vi "Waveform Analysis (Polling).vi"() -> ()   [LabVIEW 2012]
uses:
  <vilib>/Analysis/2dsp.llb/Real FFT.vi
  <vilib>/Analysis/NI_AALPro.lvlib
panel:
  out "频谱":dbl[](graph)
  out "最小值":dbl
  out "最大值":dbl
  out "时间序列":dbl[](graph)
  in  "获取最大值与最小值":bool
  in  "计算FFT":bool
  in  "获取时间序列":bool
  in  "Stop":bool
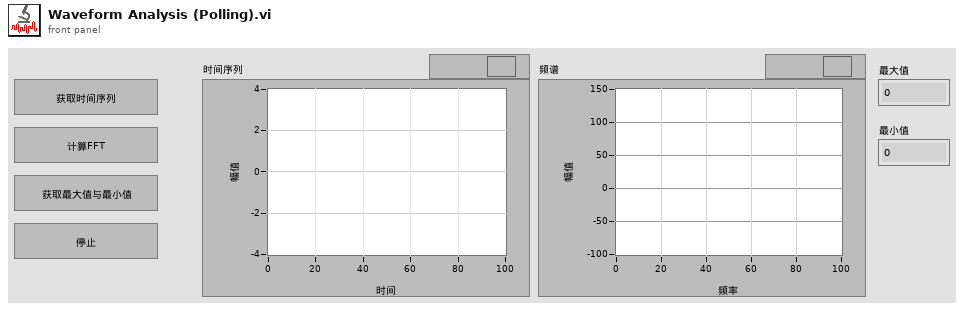
[diagram p1: front panel]
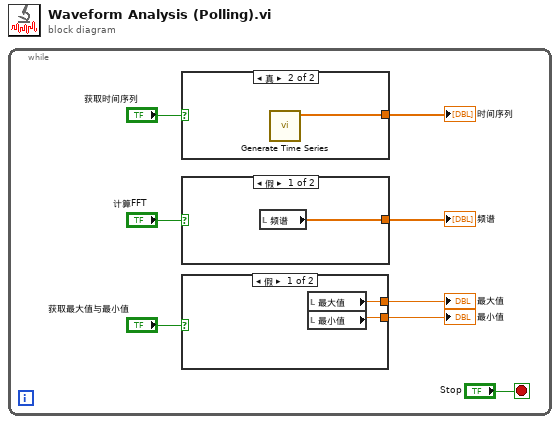
[diagram p0: block diagram]
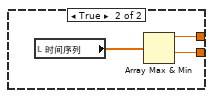
[diagram p2: hidden frame]
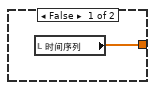
[diagram p3: hidden frame]
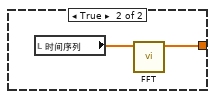
[diagram p4: hidden frame]
diagram:
  n1 = while {
    stop <- "Stop" stop-if-true
    n2 = case shown="真" "获取时间序列" {
      tunnel: [w14 w15] -> w4
      frame False {
        n3 = local read "时间序列"() -> (w14:dbl[])
      }
      frame True {
        n4 = call "Generate Time Series.vi"() -> ("时间序列"=w15:dbl[])  [unwired: 11 in]
      }
    }
    "时间序列" <- w4
    n5 = case shown="假" "计算FFT" {
      tunnel: [w16 w17] -> w1
      frame False {
        n6 = local read "频谱"() -> (w16:dbl[])
      }
      frame True {
        n7 = local read "时间序列"() -> (w18:dbl[])
        n8 = call-poly <vilib>:"FFT.vi"("X"=w18) -> ("FFT {X}"=w17:cdb[])  [unwired: 9 in, 1 out]
      }
    }
    "频谱" <- w1
    n9 = case shown="假" "获取最大值与最小值" {
      tunnel: [w10 w12] -> w3
      tunnel: [w9 w11] -> w2
      frame False {
        n10 = local read "最大值"() -> (w10:dbl)
        n11 = local read "最小值"() -> (w9:dbl)
      }
      frame True {
        n12 = local read "时间序列"() -> (w13:dbl[])
        n13 = Array Max & Min ("数组最大值与最小值")(array=w13) -> (max value=w12:dbl, min value=w11:dbl)  [unwired: 2 out]
      }
    }
    "最大值" <- w3
    "最小值" <- w2
  }
